vi "Destroy.vi"(8 "error in (no error)":errorcluster, 11 "Texture in":refnum<class "Texture.lvclass">) -> (0 "error out":errorcluster)   [LabVIEW 2021, in "Texture.lvclass"]
uses:
  Texture.lvclass
  Texture.lvclass/Texture.ctl
  LabSDL2/Source/Libraries/LibSDL2 Wrapper/LibSDL2.lvlib
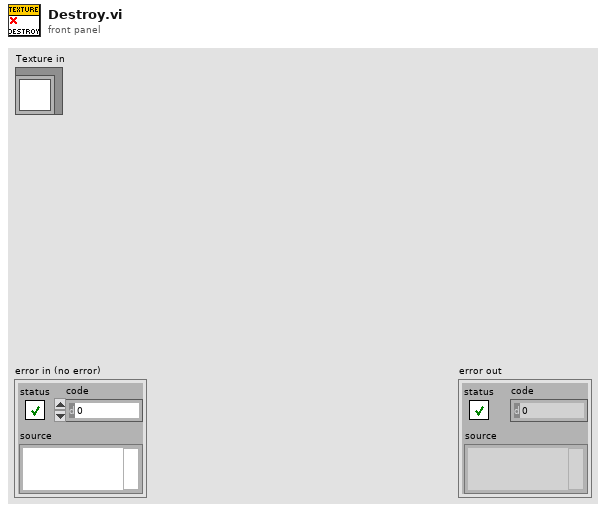
[diagram p1: front panel]
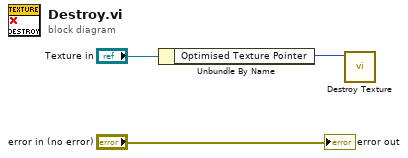
[diagram p0: block diagram]
diagram:
  n1 = Unbundle By Name("Texture in") -> ("Optimised Texture Pointer"=w1:u32)
  n2 = call "Destroy Texture.vi"("Texture Pointer"=w1) -> ()  [unwired: 10 in, 1 out]
  "error out" <- "error in (no error)"
